vi "Send Pre-Addressed Unsubscribe.vi"(8 "error in (no error)":errorcluster, 10 "SubscriptionPolicy":T1, 11 "Unsubscribe Msg In":refnum<class "Unsubscribe Msg.lvclass">) -> (0 "error out":errorcluster)   [LabVIEW 2020, in "IMediator.lvlib" / "Unsubscribe Msg.lvclass"]
doc: "发送取消订阅消息"
uses:
  Unsubscribe Msg.lvclass
  ISubscriptionPolicy/ISubscriptionPolicy Reference.ctl
  ISubscriptionPolicy/ISubscriptionPolicy.lvclass
  Unsubscribe Msg.lvclass/Unsubscribe Msg.ctl
  composed-af-messages/Source/RoundTripMessage/RoundTripMessage.lvclass/RoundTripMessage.ctl
  <vilib>/ActorFramework/Message Enqueuer/Message Enqueuer.lvclass/Message Enqueuer.ctl
  <vilib>/ActorFramework/Message Enqueuer/Enqueue.vi
  composed-af-messages/Source/RoundTripMessage/RoundTripMessage.lvclass
  C:/Program Files/National Instruments/LabVIEW 2020/vi.lib/ActorFramework/Message/Message.lvclass
  <vilib>/ActorFramework/Message Priority Queue/Priority Enqueue.vi
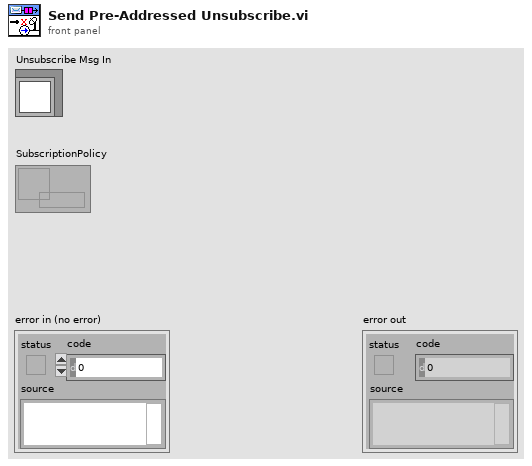
[diagram p1: front panel]
types:
  T1 = typedef "IMediator.lvlib/ISubscriptionPolicy.lvclass/ISubscriptionPolicy Reference.ctl" = refnum<data-value>
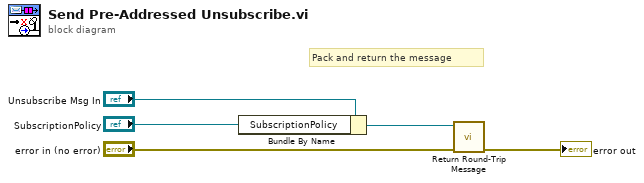
[diagram p0: block diagram]
diagram:
  # "Pack and return the message"
  n1 = Bundle By Name(cluster="Unsubscribe Msg In", "SubscriptionPolicy"="SubscriptionPolicy") -> (w3:refnum<class "Unsubscribe Msg.lvclass">)
  n2 = call "Return Round-Trip Message.vi"("error in (no error)"="error in (no error)", "RoundTripMessage In"=w3) -> ("error out"=→"error out":errorcluster)  [unwired: 9 in]
